vi "error_code_5005_element_type_not_supported.vi"(8 "error in (no error)":errorcluster, 11 "name":string) -> (0 "error out":errorcluster)   [LabVIEW 2015, in "BSON_convertors_Library.lvlib"]
doc: "Created by Artem Shevelev\nLabVIEW Portal profile: http://www.labviewportal.org/memberlist.php?mode=viewprofile&u=2340\ne-mail: artem.sh@gmail.com\nshevelev.pro"
uses:
  BSON_convertors_Library.lvlib
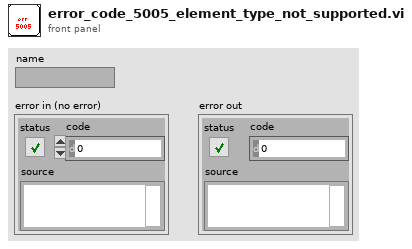
[diagram p1: front panel]
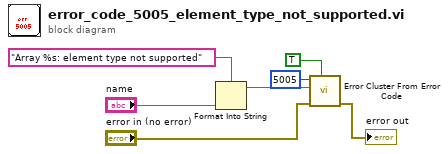
[diagram p0: block diagram]
diagram:
  n1 = Format Into String(format string="Array %s: element type not supported", "name") -> (resulting string=w3:string)  [unwired: 2 in, 1 out]
  n2 = call <vilib>:"Error Cluster From Error Code.vi"("show call chain? (False)"=TRUE, "error in (no error)"="error in (no error)", "error message (\"\")"=w3, "error code (0)"=5005) -> ("error out"=→"error out":errorcluster)  [unwired: 5 in]
